vi "Rcv Cmd.vi"(8 "error in":errorcluster, 11 "PAS in":refnum<class "PAS.lvclass">) -> (0 "error out":errorcluster, 3 "PAS out":refnum<class "PAS.lvclass">)   [LabVIEW 2016, in "PAS Library.lvlib" / "PAS.lvclass"]
doc: "The override of the <b>Instrument:Rcv Cmd</b> method accounts for checking for speaker switching when the object is set to autocycle. How the change in switch state is executed is left to the <b>Change Speaker State</b> command object which is sent when the state is to be changed."
uses:
  PAS.lvclass
  G:/sw_repo/For Builds/Reusable/Instrument/Instrument.lvclass
  Instrument/Instrument.lvclass/Instrument.ctl
  Cell/PAS Cell.lvclass/PAS Cell.ctl
  Cell/Read speaker.vi
  Cell/Read Mod Freq.vi
  Instrument/Read ExtCom.vi
  Read Cells.vi
  Cell/PAS Cell.lvclass
  Instrument/Instrument.lvclass
  Switch/Switch.lvclass
  Commands/Change Speaker State CMD/Change Speaker State CMD.lvclass
  G:/sw_repo/For Builds/Reusable/Command/Command.lvclass
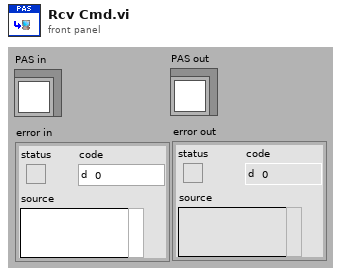
[diagram p1: front panel]
types:
  T1 = cluster{"tag":string, "section":string, "data":variant}
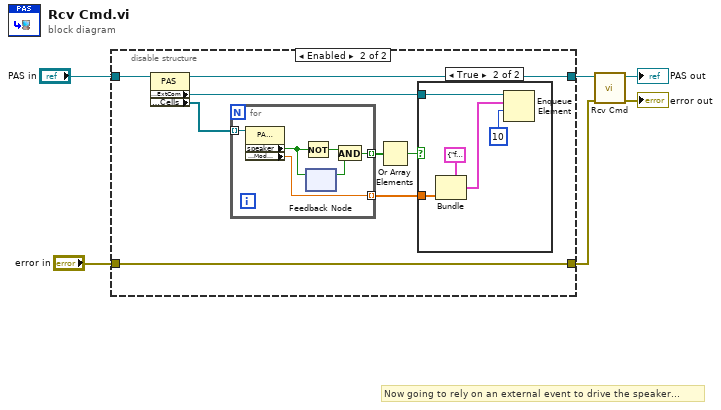
[diagram p0: block diagram]
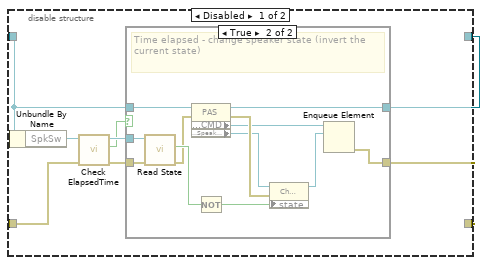
[diagram p2: hidden frame]
diagram:
  # "Now going to rely on an external event to drive the speaker..."
  n1 = disable-structure shown="Enabled" {
    disable-tunnel: "PAS in" -> [w10 w36]
    disable-tunnel: [w9 w30] -> w3
    disable-tunnel: [w8 w29] -> w2
    disable-tunnel: "error in" -> [w7 w29]
    frame Disabled {
      n2 = Unbundle By Name(w10) -> ("SpkSw"=w14:refnum<class "Switch.lvclass">)
      n3 = call-dynamic "Check ElapsedTime.vi"("error in"=w7, "Switch in"=w14) -> ("error out"=w12:errorcluster, "Cycle Switch?"=w11:bool, "Switch out"=w13:refnum<class "Switch.lvclass">)  [unwired: 6 in, 1 out]
      n4 = case shown="True" w11 {
        tunnel: w13 -> [_ w28]
        tunnel: w12 -> [w15 w27]
        tunnel: w10 -> [w16 w25]
        tunnel: [w16 w19] -> w9
        tunnel: [w15 w18] -> w8
        frame False {
        }
        frame True {
          # "Time elapsed - change speaker state (invert the current state)"
          n5 = call-dynamic "Read State.vi"("error in (no error)"=w27, "Switch in"=w28) -> ("error out"=w24:errorcluster, "State"=w26:bool)  [unwired: 7 in, 1 out]
          n6 = property class="PAS"(reference=w25, error in=w24) -> (reference out=w19:refnum<class "PAS.lvclass">, error out=w22:errorcluster, "Accessors:CMD"=w20:refnum<queue>, "Data Access:Speaker State CMD"=w17:refnum<class "Change Speaker State CMD.lvclass">)
          n7 = Not(x=w26) -> (.not. x?=w23:bool)
          n8 = property class="Change Speaker State CMD"(reference=w17, error in=w22, "state"=w23) -> (reference out=w21:refnum<class "Change Speaker State CMD.lvclass">)  [unwired: 1 out]
          n9 = Enqueue Element(queue=w20, element=w21) -> (error out=w18:errorcluster)  [unwired: 2 in, 2 out]
        }
      }
    }
    frame Enabled {
      n10 = property class="PAS"(reference=w36) -> (reference out=w30:refnum<class "PAS.lvclass">, "Accessors:ExtCom"=w35:refnum<queue>, "Data Access:Cells"=w34:refnum<class "PAS Cell.lvclass">[])  [unwired: 1 in, 1 out]
      n11 = for {
        tunnel: w34 -> [w47] mode=indexing
        tunnel: [w43] -> w33 mode=indexing
        tunnel: [w42] -> w32 mode=indexing
        n12 = property class="PAS Cell"(reference=w47) -> ("speaker"=w46:bool, "Accessors:Mod Freq"=w43:sgl)  [unwired: 1 in, 2 out]
        n13 = Not(x=w46) -> (.not. x?=w44:bool)
        n14 = feedback-in #1(w46) -> ()
        n15 = feedback #1() -> (w45:bool)  [unwired: 1 in]
        n16 = And(x=w44, y=w45) -> (x .and. y?=w42:bool)
      }
      n17 = Or Array Elements(Boolean array=w32) -> (logical OR=w31:bool)
      n18 = case shown="True" w31 {
        tunnel: w35 -> [_ w41]
        tunnel: w33 -> [_ w39]
        frame False {
        }
        frame True {
          n19 = Bundle(cluster=T1 {"tag"="fmod", "section"="pas", "data"=variant} ("element"), "data"=w39) -> (w38:T1)  [unwired: 2 in]
          n20 = Enqueue Element(queue=w41, element=w38, timeout in ms (-1)=10) -> ()  [unwired: 1 in, 3 out]
        }
      }
    }
  }
  n21 = call-parent "Rcv Cmd.vi"("error in"=w2, "Instrument in"=w3) -> ("error out"=→"error out":errorcluster, "Instrument out"=→"PAS out":refnum<class "PAS.lvclass">)  [unwired: 8 in]
